vi "Process-Logging.vi"(9 "Wait on post-processing":refnum<k4>, 10 "Queues Cluster":T1, 11 "Data-gen queue":T2) -> (0 "error out":errorcluster)   [LabVIEW 2017]
uses:
  Logging/Typedefs/ROI File Generator Queue Ref.ctl
  Typedefs/Logging queue element.ctl
  Typedefs/Imaging Protocols enum.ctl
  Typedefs/Frame Size.ctl
  Typedefs/Acquired points count.ctl
  User Interface/Queue/Message Queue/Typedefs/All Message Queues.ctl
  User Interface/Queue/Message Queue/Typedefs/Message Cluster.ctl
panel:
  out "Loop iterations":i32
  out "Number of trials closed":u32
  out "Loop period (ms)":u32
  # "TIME-CRITICAL MODULE"
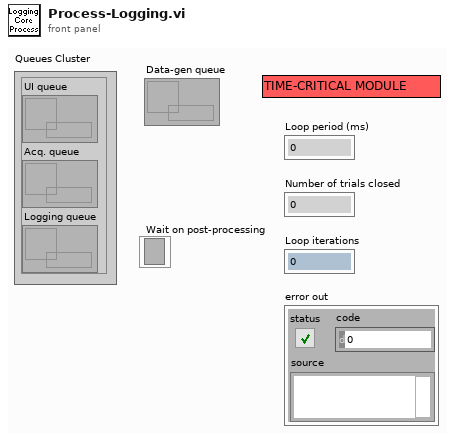
[diagram p1: front panel]
types:
  T1 = typedef "All Message Queues.ctl" = cluster{"UI queue":refnum<queue>, "Acq. queue":refnum<queue>, "Logging queue":refnum<queue>}
  T2 = typedef "ROI File Generator Queue Ref.ctl" = refnum<queue>
  T3 = cluster{"TDMS group name":string, "TDMS channel names array":string[]}
  T4 = typedef "Live graph data queue ref.ctl" = refnum<queue>
  T5 = typedef "Live imaging queue element.ctl" = cluster{"Red channel":T6, "Green channel":T6, "Ref Red channel":T6, "Ref Green channel":T6, "Mov cor":bool}
  T6 = typedef "IMAQ Image.ctl" = refnum<image>
  T7 = typedef "Logging queue element.ctl" = cluster{"Imaging Protocol":T8, "Number of Trials":u16, "Frame Size":T9, "# Averaged frames":u16, "Dwell time (us)":dbl, "Index of Z-plane":i32, "Timelapse?":bool, "Logging process is active":bool, "Speed logging enabled":bool, "tdms file ref":refnum<k34>, "path":path, "Trial Number":i32, "Expected # points acquired":bool, "Manually stopped":bool, "Last trial":bool, "Ch0 data":u32[], "Ch1 data":u32[], "Image Time":u64[], "Continuous Time":u64[], "Points acquired":T10, "HW Timings File":refnum<file>}
  T8 = typedef "Imaging Protocols enum.ctl" = enum16{"AOL Z-Stack", "Motor Z Stack", "Functional Acquisition", "Single Plane Acquisition", "Volume Acquisition", "Live Imaging", "Live Plane Imaging", "Live Volume Imaging"}
  T9 = typedef "Frame Size.ctl" = u16
  T10 = typedef "Acquired points count.ctl" = cluster{"Ch0 last trial":u64, "Ch1 last trial":u64, "All trials":u64}
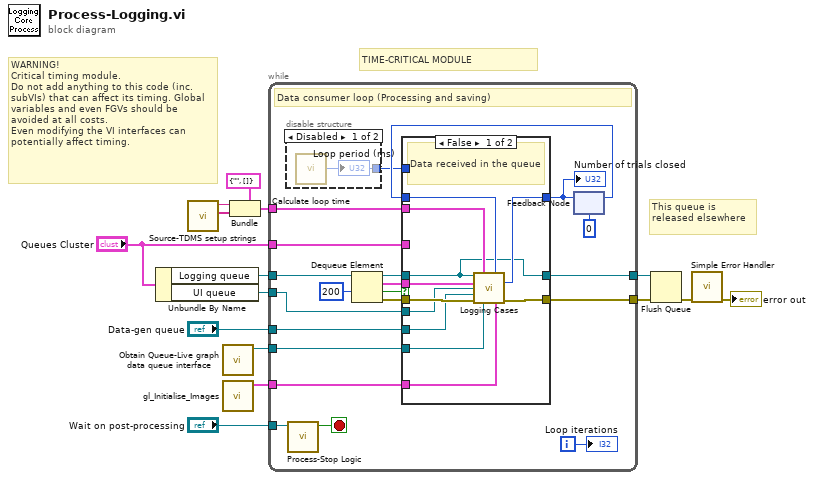
[diagram p0: block diagram]
diagram:
  # "WARNING!\nCritical timing module.\nDo not add anything to this code (inc. subVIs) that can affect its timing. Global variables and even FGVs should be avoided at all costs.\nEven modifying the VI interfaces can potentially affect timing."
  # "TIME-CRITICAL MODULE"
  # "This queue is released elsewhere"
  n1 = Unbundle By Name("Queues Cluster") -> ("Logging queue"=w3:refnum<queue>, "UI queue"=w1:refnum<queue>)
  n2 = call "Source-TDMS setup strings.vi"() -> ("Functional imaging TDMS channel names array"=w5:string[], "TDMS group name"=w6:string)  [unwired: 10 in]
  n3 = call "Obtain Queue-Live graph data queue interface.vi"() -> ("Live graphs queue"=w13:T4)  [unwired: 10 in, 1 out]
  n4 = call "gl_Initialise_Images.vi"() -> ("Live image refs"=w12:T5)  [unwired: 11 in]
  n5 = Bundle(cluster=T3 {"TDMS group name"="", "TDMS channel names array"=[]} ("Channel info"), "TDMS group name"=w6, "TDMS channel names array"=w5) -> (w4:T3)
  n6 = while {
    tunnel: [w33] -> w8
    tunnel: "Data-gen queue" -> [w31]
    tunnel: w12 -> [w29]
    tunnel: w13 -> [w27]
    tunnel: w3 -> [w32]
    tunnel: [w19] -> w9
    tunnel: "Wait on post-processing" -> [w20]
    tunnel: w4 -> [w22]
    tunnel: "Queues Cluster" -> [w18]
    tunnel: w1 -> [w17]
    i -> [w28]
    stop <- w21 stop-if-true
    # "Data consumer loop (Processing and saving)"
    n7 = disable-structure shown="Disabled" {
      disable-tunnel: [w37 _] -> w23
      frame Disabled {
        n8 = call <userlib>:"Calculate loop time.vi"() -> ("Loop time (ms)"=w37:u32)  [unwired: 11 in]
        "Loop period (ms)" <- w37
      }
      frame Enabled {
      }
    }
    n9 = call "Process-Stop Logic.vi"("Wait on post-processing"=w20) -> ("Abort logging"=w21:bool)  [unwired: 10 in]
    n10 = Dequeue Element(queue=w32, timeout in ms (-1)=200) -> (queue out=w16:refnum<queue>, element=w35:T7, timed out?=w26:bool, error out=w36:errorcluster)  [unwired: 1 in]
    n11 = feedback #1(u32 0 ("Number of files closed")) -> (w30:u32)
    n12 = case shown="False" w26 {
      tunnel: [w48 w51] -> w33
      tunnel: w36 -> [w47 w51]
      tunnel: w35 -> [w45 _]
      tunnel: w31 -> [w46 _]
      tunnel: [w40 w50] -> w25
      tunnel: w30 -> [w41 w50]
      tunnel: w29 -> [w43 _]
      tunnel: w27 -> [w44 _]
      tunnel: w16 -> [w39 w49]
      tunnel: w23 -> [_ _]
      tunnel: w22 -> [w42 _]
      tunnel: [w39 w49] -> w19
      tunnel: w18 -> [_ _]
      tunnel: w17 -> [w38 _]
      frame False {
        # "Data received in the queue"
        n13 = call "Logging Cases.vi"("Logging queue"=w39, "Channel info"=w42, "Number of files closed in"=w41, "Logging queue element in"=w45, "UI queue"=w38, "Data-gen queue"=w46, "error in"=w47, "Live graph data queue in"=w44, "Image array"=w43) -> ("Number of TDMS files closed"=w40:u32, "error out"=w48:errorcluster)  [unwired: 5 in]
      }
      frame True {
        # "Timed out (200ms). This case allows stopping the loop correctly."
      }
    }
    "Number of trials closed" <- w25
    n14 = feedback-in #1(w25) -> ()
    "Loop iterations" <- w28
  }
  n15 = Flush Queue(queue=w9, error in (no error)=w8) -> (error out=w10:errorcluster)  [unwired: 2 out]
  n16 = call <vilib>:"Simple Error Handler.vi"("error in (no error)"=w10) -> ("error out"=→"error out":errorcluster)  [unwired: 4 in, 4 out]
